vi "Draw Number Array.vi"(8 "Error In":errorcluster, 10 "Number of Mines Array":u32[][](array[numeric]), 11 "Picture In":picture) -> (0 "Error Out":errorcluster, 3 "Picture Out":picture)   [LabVIEW 2011]
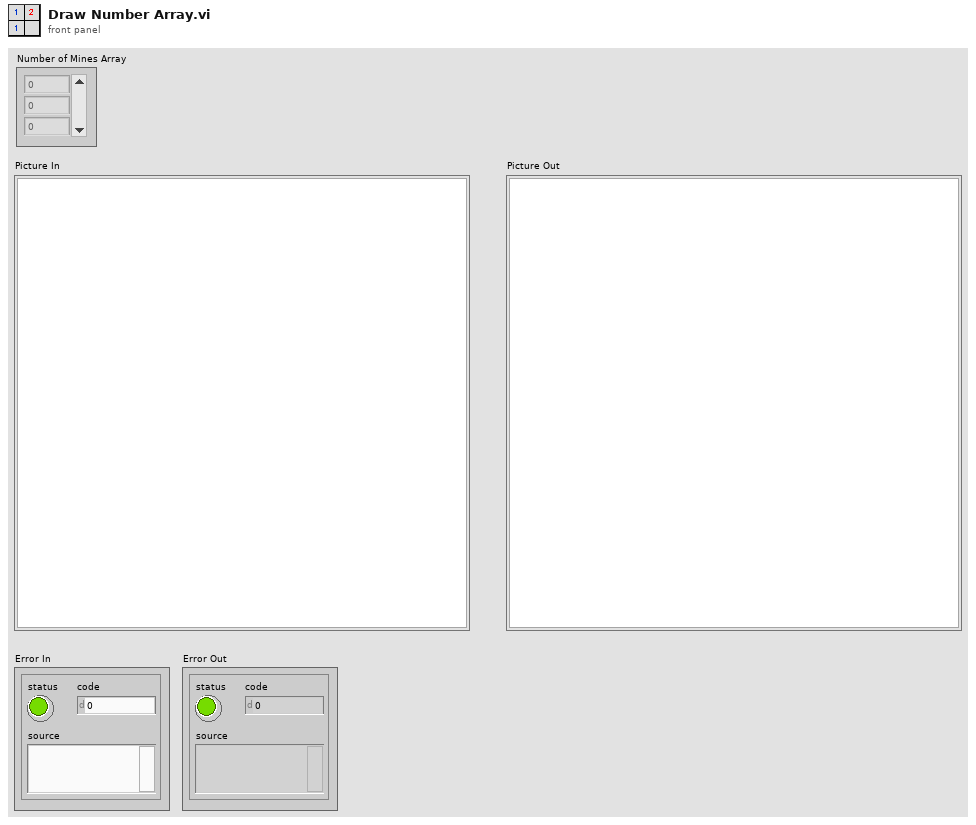
[diagram p1: front panel]
types:
  T1 = enum16{"User-specified Font", "Application Font", "System Font", "Dialog Font"}
  T2 = cluster{"Font Name:":string, "Size":i16, "Strikeout?":bool, "Italic?":bool, "Underline?":bool, "Outline?":bool, "Shadow?":bool, "Bold?":bool}
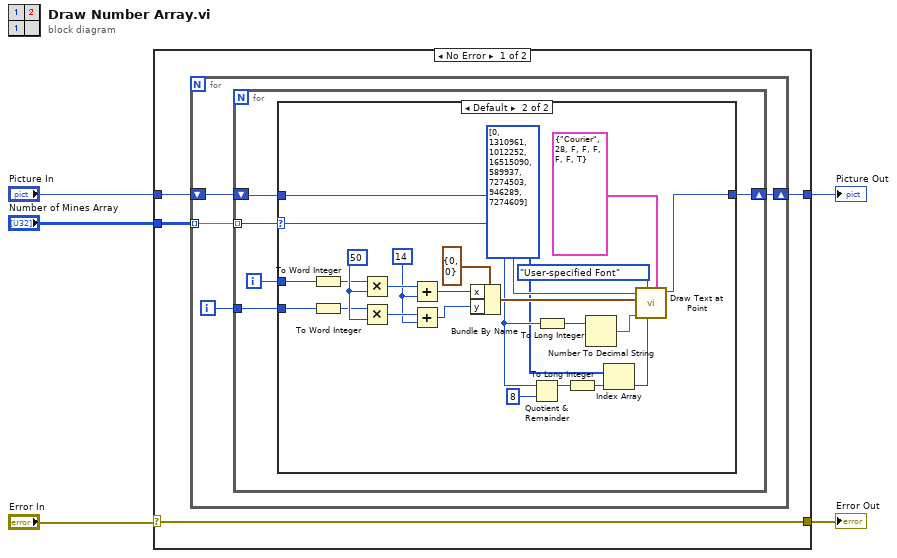
[diagram p0: block diagram]
diagram:
  n1 = case shown="No Error" "Error In" {
    selector: "Error In" -> [w6 w44]
    tunnel: "Picture In" -> [w9 w45]
    tunnel: "Number of Mines Array" -> [w8 _]
    tunnel: [w7 w45] -> w3
    tunnel: [w6 w44] -> w1
    frame No Error {
      n2 = for {
        tunnel: w8 -> [w11] mode=indexing
        shift-right: [w10] -> w7
        shift-left: w9 -> [w13]
        i -> [w12]
        n3 = for {
          tunnel: w12 -> [w16]
          tunnel: w11 -> [w14] mode=indexing
          shift-right: [w15] -> w10
          shift-left: w13 -> [w18]
          i -> [w17]
          n4 = case shown="Default" w14 {
            selector: w14 -> [_ w25]
            tunnel: w18 -> [w19 w43]
            tunnel: w17 -> [_ w35]
            tunnel: w16 -> [_ w33]
            tunnel: [w19 w30] -> w15
            frame 0 {
            }
            frame Default {
              w38 = i16 14
              w41 = i16 50
              n5 = To Word Integer(number=w35) -> (16bit integer=w34:i16)
              n6 = To Word Integer(number=w33) -> (16bit integer=w32:i16)
              n7 = Multiply(x=w34, y=w41) -> (x*y=w40:i16)
              n8 = Multiply(x=w32, y=w41) -> (x*y=w39:i16)
              n9 = Add(x=w40, y=w38) -> (x+y=w37:i16)
              n10 = Add(x=w39, y=w38) -> (x+y=w36:i16)
              n11 = Bundle By Name(cluster=cluster{"x":i16, "y":i16} {"x"=0, "y"=0} ("origin"), "x"=w37, "y"=w36) -> (w31:cluster{"x":i16, "y":i16})
              n12 = Quotient & Remainder(x=w25, y=u32 8) -> (x-y*floor(x/y)=w20:u32)  [unwired: 1 out]
              n13 = To Long Integer(number=w25) -> (32bit integer=w26:i32)
              n14 = To Long Integer(number=w20) -> (32bit integer=w21:i32)
              n15 = Number To Decimal String(number=w26) -> (decimal integer string=w27:string)  [unwired: 1 in]
              n16 = Index Array(array=u32[] [0, 1310961, 1012252, 16515090, 589937, 7274503, 946289, 7274609], index=w21) -> (element=w22:u32)
              n17 = call <vilib>:"Draw Text at Point.vi"("[user-specified font]"=T2 {"Font Name:"="Courier", "Size"=28, "Strikeout?"=FALSE, "Italic?"=FALSE, "Underline?"=FALSE, "Outline?"=FALSE, "Shadow?"=FALSE, "Bold?"=TRUE}, "text color(black)"=w22, "desired font(Application)"=T1."User-specified Font", "text"=w27, "origin"=w31, "picture"=w43) -> ("new picture"=w30:picture)  [unwired: 4 in, 1 out]
            }
          }
        }
      }
    }
    frame Error {
    }
  }
  "Picture Out" <- w3
  "Error Out" <- w1
